vi "Configure Timer.vi"(0 "VISA resource name":refnum<visa-resource-name>, 1 "Channel (1:CH1)":u16(ring)=1 items=["CH1"=1, "CH2"=2], 5 "Voltage (0 V)":dbl min=0.0 max=32.0 format="%.3f", 7 "Current (0 A)":dbl min=0.0 max=3.2 format="%.3f", 9 "Duration (0 s)":dbl min=0.0 max=10000.0 step=1.0, 11 "error in (no error)":errorcluster, 12 "Group Number (1:1)":u16(ring)=1 items=["1"=1, "2"=2, "3"=3, "4"=4, "5"=5]) -> (4 "VISA resource name out":refnum<visa-resource-name>, 15 "error out":errorcluster)   [LabVIEW 2015, in "Siglent SPD3000 Series.lvlib"]
doc: "Configures the timer function.\n\n<B>Note:</B>\nThis VI is invalid for the SPD3303C models."
uses:
  <instrlib>/Siglent SPD3000 Series/Siglent SPD3000 Series.lvlib
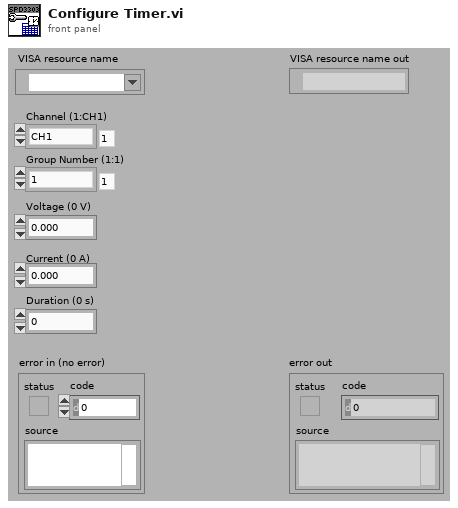
[diagram p1: front panel]
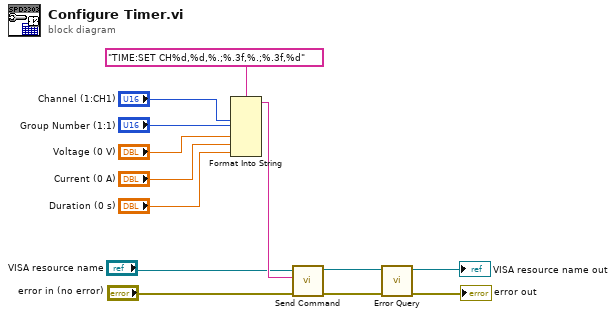
[diagram p0: block diagram]
diagram:
  n1 = Format Into String(format string="TIME:SET CH%d,%d,%.;%.3f,%.;%.3f,%d" ("写入缓冲区"), "Channel (1:CH1)", "Group Number (1:1)", "Voltage (0 V)", "Current (0 A)", "Duration (0 s)") -> (resulting string=w3:string)  [unwired: 2 in, 1 out]
  n2 = call <instrlib>:"Send Command.vi"("error in (no error)"="error in (no error)", "Write Buffer (\"\")"=w3, "VISA resource name"="VISA resource name") -> ("error out"=w4:errorcluster, "VISA resource name out"=w5:refnum<visa-resource-name>)  [unwired: 7 in]
  n3 = call <instrlib>:"Error Query.vi"("error in (no error)"=w4, "VISA resource name"=w5) -> ("error out"=→"error out":errorcluster, "VISA resource name out"=→"VISA resource name out":refnum<visa-resource-name>)  [unwired: 6 in, 2 out]
